vi "KM101_MoveRelativeStep.vi"(8 "bWait":bool, 9 "RelSteps":i32, 10 "Channel":i32, 11 "reference in":refnum<k7>) -> (2 "reference out":refnum<k7>)   [LabVIEW 2018, in "KIM101lib.lvlib"]
uses:
  KIM101lib.lvlib
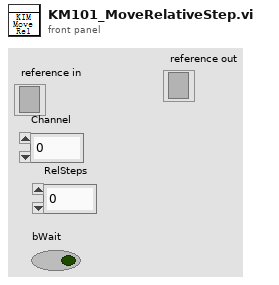
[diagram p1: front panel]
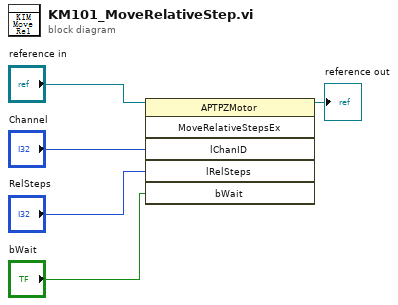
[diagram p0: block diagram]
diagram:
  n1 = invoke class="APTPZMotor" method="MoveRelativeStepsEx"(reference="reference in", "lChanID"="Channel", "lRelSteps"="RelSteps", "bWait"="bWait") -> (reference out=→"reference out":refnum<k7>)  [unwired: 2 in, 5 out]
